vi "SetSpeed2.vi"(11 "Chaîne en entrée":string) -> ()   [LabVIEW 2015]
uses:
  <vilib>/myRIO/Instrument Drivers/Onboard IO/UART/typedef/VISA Configuration.ctl
  <vilib>/Instr/_visa.llb/VISA Configure Serial Port (Instr).vi
  <vilib>/myRIO/Express VI/Onboard IO/UART/UART Express VI.xnode
  <vilib>/myRIO/Instrument Drivers/Onboard IO/UART/UART.lvlib
panel:
  in  "error in (no error)":errorcluster
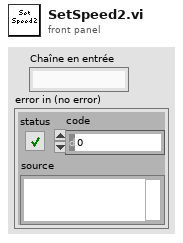
[diagram p1: front panel]
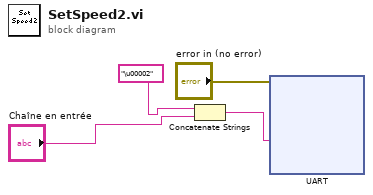
[diagram p0: block diagram]
diagram:
  n1 = Concatenate Strings("\u00002", "Chaîne en entrée") -> (w2:string)
  n2 = xnode "UART"("Characters to Write"=w2, "error in (no error)"="error in (no error)") -> ()  [unwired: 2 out]
